vi "AddTriggeredEventsToStates.vi"(0 "State Array In":string[](array[string]), 2 "Event List":string[](array[string]), 4 "Event Triggers Array":bool[](array[boolean])) -> (14 "State Array Out":string[](array[string]))   [LabVIEW 2011]
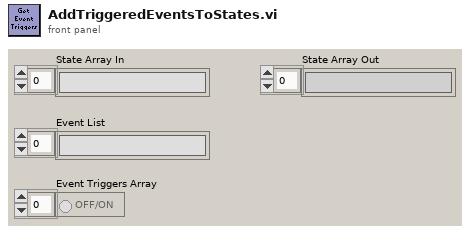
[diagram p1: front panel]
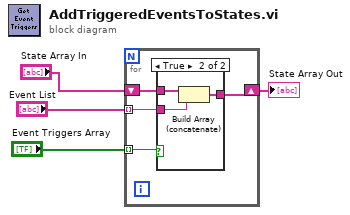
[diagram p0: block diagram]
diagram:
  n1 = for {
    tunnel: "Event List" -> [w7] mode=indexing
    tunnel: "Event Triggers Array" -> [w8] mode=indexing
    shift-right: [w5] -> w3
    shift-left: "State Array In" -> [w6]
    n2 = case shown="True" w8 {
      tunnel: w7 -> [_ w11]
      tunnel: w6 -> [w9 w12]
      tunnel: [w9 w10] -> w5
      frame False {
      }
      frame True {
        n3 = Build Array (concatenate)(w12, w11) -> (w10:string[])
      }
    }
  }
  "State Array Out" <- w3
